vi "Command DriveDistanceAtAngle.vi"() -> (0 "Reinit":bool)   [LabVIEW 2019]
uses:
  Old Code/M14_Robot_Code/Robot_Code/Auto/Auto Utilities/Command_Execution_State.ctl
panel:
  in  "Numeric 3":dbl
  in  "Numeric 2":dbl
  in  "Numeric":dbl
  out "Completed":bool
  in  "Startup":bool
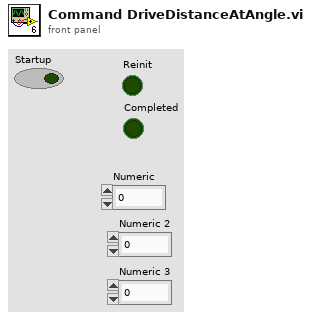
[diagram p1: front panel]
types:
  T1 = typedef "Command_Execution_State.ctl" = enum16{"Initialize", "Execute", "Finish"}
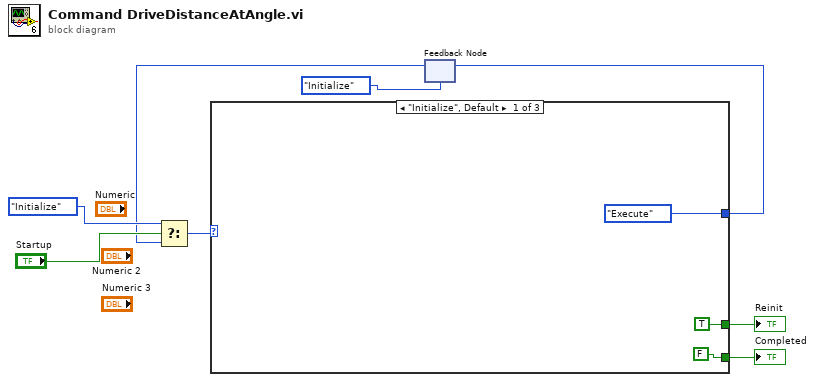
[diagram p0: block diagram]
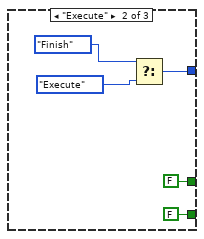
[diagram p2: hidden frame]
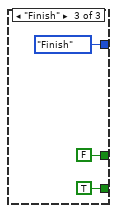
[diagram p3: hidden frame]
diagram:
  n1 = feedback #1(Command_Execution_State."Initialize") -> (w4:T1)
  n2 = Select(t=Command_Execution_State."Initialize", s="Startup", f=w4) -> (s? t:f=w6:T1)
  n3 = case shown="\"Initialize\", Default" w6 {
    tunnel: [Command_Execution_State."Execute" w14 Command_Execution_State."Finish"] -> w5
    tunnel: [TRUE ("Reinit") FALSE ("Reinit") FALSE ("Reinit")] -> w2
    tunnel: [FALSE ("Reinit") FALSE ("Reinit") TRUE ("Reinit")] -> w1
    frame "Initialize", Default {
    }
    frame "Execute" {
      n4 = Select(t=Command_Execution_State."Finish", f=Command_Execution_State."Execute") -> (s? t:f=w14:T1)  [unwired: 1 in]
    }
    frame "Finish" {
    }
  }
  "Reinit" <- w2
  "Completed" <- w1
  n5 = feedback-in #1(w5) -> ()
